vi "GetItem.vi"(8 "Error":errorcluster, 10 "Tag":string, 11 "Tree in":refnum<class "Tree.lvclass">) -> (0 "Error":errorcluster, 2 "ItemData":T1, 3 "Tree out":refnum<class "Tree.lvclass">)   [LabVIEW 2021, in "Tree.lvlib" / "Tree.lvclass"]
uses:
  Tree.lvclass
  Private/TreeControllerTag.ctl
  Tree.lvclass/Tree.ctl
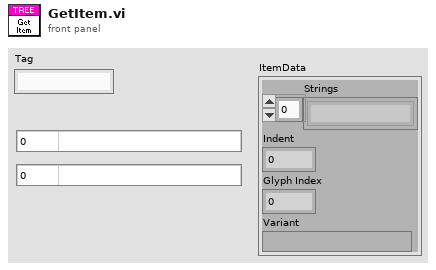
[diagram p1: front panel]
types:
  T1 = cluster{"Strings":string[], "Indent":i32, "Glyph Index":i32, "Variant":variant}
  T2 = typedef "Tree.lvlib/Tree.lvclass/TreeControllerTag.ctl" = enum8{"Null", "1. Add item", "2. Delete item", "3. Get All Tree Data", "4. Drag Starting", "5. Drag Ended", "6. Add Tree Values", "7. Get Item Value", "8. Edit Item", "9. StepBack", "10. Filter"}
  T3 = cluster{string[], "Item Indent":i32, "Glyph Index":i32, "Value":variant}
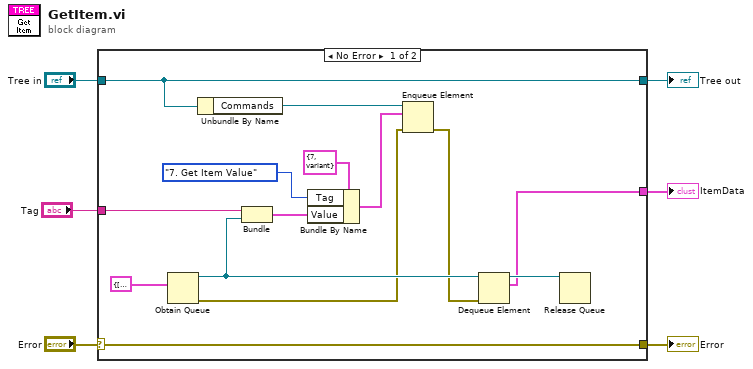
[diagram p0: block diagram]
diagram:
  n1 = case shown="No Error" "Error" {
    selector: "Error" -> [w20 w22]
    tunnel: [w20 w22] -> w5
    tunnel: [w10 w21] -> w3
    tunnel: "Tree in" -> [w10 w21]
    tunnel: "Tag" -> [w16 _]
    tunnel: [w8 _] -> w1
    frame No Error {
      n2 = Obtain Queue(element data type=T3 {[], "Item Indent"=0, "Glyph Index"=0, "Value"=variant} ("output cluster")) -> (queue out=w13:refnum<queue>, error out=w12:errorcluster)  [unwired: 4 in, 1 out]
      n3 = Unbundle By Name(w10) -> ("Commands"=w19:refnum<queue>)
      n4 = Bundle("Tag"=w16, "queue out"=w13) -> (w14:cluster{"Tag":string, "queue out":refnum<queue>})  [unwired: 1 in]
      n5 = Bundle By Name(cluster=cluster{"Tag":u8, "Value":variant} {"Tag"=7, "Value"=variant} ("element"), "Tag"=TreeControllerTag."7. Get Item Value", "Value"=w14) -> (w17:cluster{"Tag":u8, "Value":variant})
      n6 = Enqueue Element(queue=w19, element=w17, error in (no error)=w12) -> (error out=w11:errorcluster)  [unwired: 1 in, 2 out]
      n7 = Dequeue Element(queue=w13, error in (no error)=w11) -> (queue out=w15:refnum<queue>, element=w8:T3)  [unwired: 1 in, 2 out]
      n8 = Release Queue(queue=w15) -> ()  [unwired: 2 in, 3 out]
    }
    frame Error {
    }
  }
  "Error" <- w5
  "Tree out" <- w3
  "ItemData" <- w1
